vi "GT Modify Password.vi"(8 "error in (no error)":errorcluster caption="错误输入（无错误）", 9 "pNewPassword":string, 10 "pOldPassword":string, 11 "cardNum":i16) -> (0 "error out":errorcluster caption="错误输出", 1 "pNewPassword out":string, 2 "pOldPassword out":string, 3 "function return":i16)   [LabVIEW 2020, in "gts1.lvlib"]
doc: "GT_API GT_ModifyPassword(short cardNum,char *pOldPassword,char *pNewPassword);"
uses:
  gts1.lvlib
  dll/32bit/multi_card/gts.dll
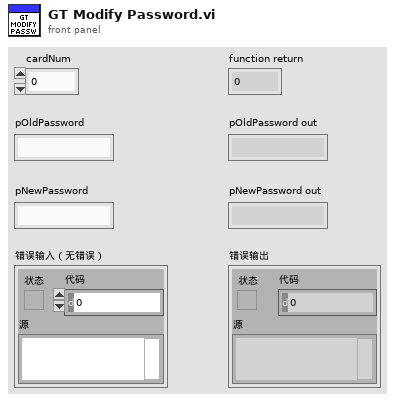
[diagram p1: front panel]
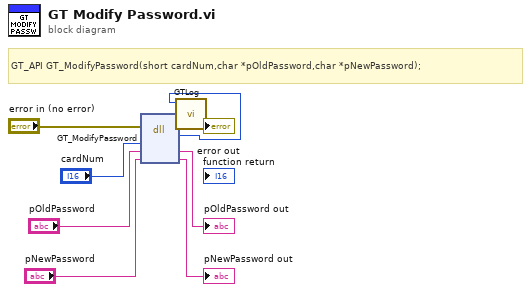
[diagram p0: block diagram]
diagram:
  # "GT_API GT_ModifyPassword(short cardNum,char *pOldPassword,char *pNewPassword);"
  n1 = dll-call lib="C:/1228/dll/32bit/multi_card/gts.dll" fn="GT_ModifyPassword"(error in="error in (no error)", "cardNum"="cardNum", "pOldPassword"="pOldPassword", "pNewPassword"="pNewPassword") -> (error out=w3:errorcluster, w1:i16, "pOldPassword"=→"pOldPassword out":string, "pNewPassword"=→"pNewPassword out":string)  [unwired: 3 in, 1 out]
  n2 = call "GTLog.vi"("error in (no error)"=w3, "Numeric"=w1) -> ("error out"=→"error out":errorcluster)  [unwired: 9 in]
